vi "lab10_target_1.vi"   [LabVIEW 2020]
uses:
  <vilib>/Platform/TimedLoop/XDataNode/timing_clust.ctl
  <vilib>/Platform/TimedLoop/XDataNode/nitl_modes.ctl
  <vilib>/Platform/TimedLoop/XDataNode/wakeup.ctl
  <vilib>/Platform/TimedLoop/scheduler/LVUserAPI/_suppVIs/Create_1MHz_TSource.vi
  <vilib>/platform/TimedLoop/XDataNode/XDataNode.xnode
  <vilib>/Platform/TimedLoop/XDataNode/XDNodeRunTimeDep.lvlib
types:
  T1 = typedef "XDNodeRunTimeDep.lvlib/timing_clust.ctl" = cluster{"Expected End [f-1]":u64, "Actual End [f-1]":u64, "Finished Late? [f-1]":bool, "Expected End [i-1]":u64, "Actual End [i-1]":u64, "Finished Late? [i-1]":bool, "Expected Start [i]":u64, "Actual Start [i]":u64, "Expected Start [f]":u64, "Actual Start [f]":u64, "Source Name":string, "Structure Name":string, "Period":i64, "Deadline":i64, "Offset":i64, "Start":i64, "Priority":i32, "Timeout":i32, "Mode":T2, "Wakeup Reason":T3, "Error":errorcluster, "Source Type":string, "Secondary Source Type":string, "Global End Time":u64, "Global Start Time":u64, "Frame Duration":u64, "Iteration Duration":u64, "Assigned CPU":i32, "I/O Scan Engine Mode":u32}
  T2 = typedef "XDNodeRunTimeDep.lvlib/nitl_modes.ctl" = enum32{"No Change", "Process missed periods, maintain original phase", "Discard missed periods, maintain original phase", "Process missed periods, ignore original phase", "Discard missed periods, ignore original phase"}
  T3 = typedef "XDNodeRunTimeDep.lvlib/wakeup.ctl" = enum32{"Normal", "Aborted", "Asynchronous wakeup", "Timing source error", "Timed loop error", "Timeout"}
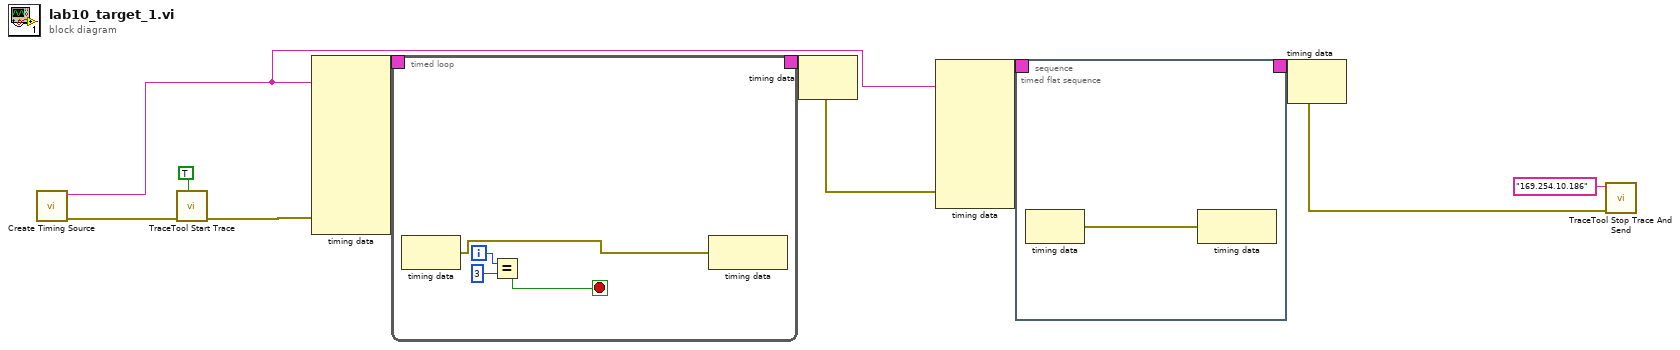
[diagram p0: block diagram]
diagram:
  n1 = call-poly <vilib>:"Create Timing Source.vi"() -> ("error out"=w6:errorcluster, "name (out)"=w1:string)  [unwired: 10 in]
  n2 = call <vilib>:"TraceTool Start Trace.vi"("Detailed Tracing? (F)"=TRUE, "error in (no error)"=w6) -> ("error out"=w5:errorcluster)  [unwired: 8 in, 1 out]
  n3 = node-c288(w1, w5) -> (w11:T1)  [unwired: 8 in]
  n4 = timed-loop {
    timing: w11 -> [_]
    timing-out: [_] -> w10
    i -> [w15]
    stop <- w13 stop-if-true
    n5 = node-c288() -> (w12:errorcluster)  [unwired: 1 in]
    n6 = Equal?(x=w15, y=3) -> (x = y?=w13:bool)
    n7 = node-c288(w12) -> ()  [unwired: 1 out]
  }
  n8 = node-c288(w10) -> (w7:errorcluster)
  n9 = node-c288(w1, w7) -> (w9:T1)  [unwired: 6 in]
  n10 = timed-sequence {
    timing: w9 -> [_]
    timing-out: [_] -> w8
    n11 = timed-flat-sequence {
      n12 = node-c288() -> (w21:errorcluster)  [unwired: 1 in]
      n13 = node-c288(w21) -> ()  [unwired: 1 out]
    }
  }
  n14 = node-c288(w8) -> (w3:errorcluster)
  n15 = call <vilib>:"TraceTool Stop Trace And Send.vi"("error in (no error)"=w3, "Trace Host Network Address"="169.254.10.186") -> ()  [unwired: 9 in, 1 out]
